vi "scanFrontPanel.vi"(8 "error in (no error)":errorcluster, 9 "index":i16, 10 "ScriptEventList":refnum<class "ScriptEventList.lvclass">, 11 "ScanCreator in":refnum<class "ScanCreator.lvclass">) -> (0 "error out":errorcluster, 1 "cancelled":bool, 2 "scriptListArray":refnum<class "ScriptEventList.lvclass">[](array[class]), 3 "ScanCreator out":refnum<class "ScanCreator.lvclass">, 4 "scanType":string, 5 "Values":string[](array[string]))   [LabVIEW 2011, in "Views.lvlib" / "ScriptEditor.lvlib" / "ScanCreator.lvclass"]
uses:
  ScanCreator.lvclass
  Tools/Scripting/ScriptingEvent/ScriptEventList/ScriptEventList.lvclass
  ScanCreator.lvclass/ScanCreator.ctl
panel:
  in  "Steps":dbl
  in  "Cancel":bool
  in  "ok":bool
  in  "Delay All?":bool=TRUE
  in  "Increment":dbl
  in  "EndValue":dbl format="%#_8g"
  in  "StartValue":dbl format="%#.8g"
  in  "Scan Type":u16(ring) items=["Time", "Time Difference", "Start Value", "End Value", "Step Value", "Ramp Time"]
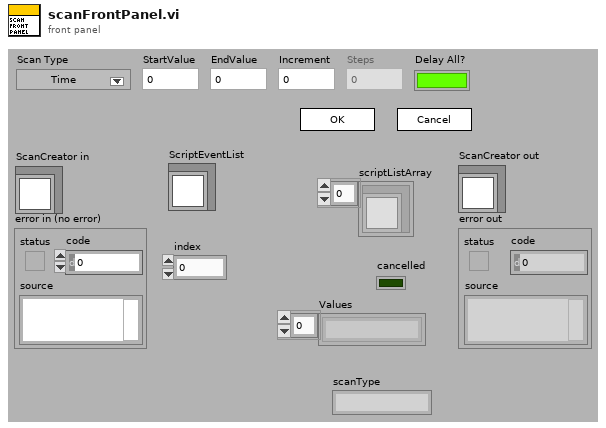
[diagram p1: front panel]
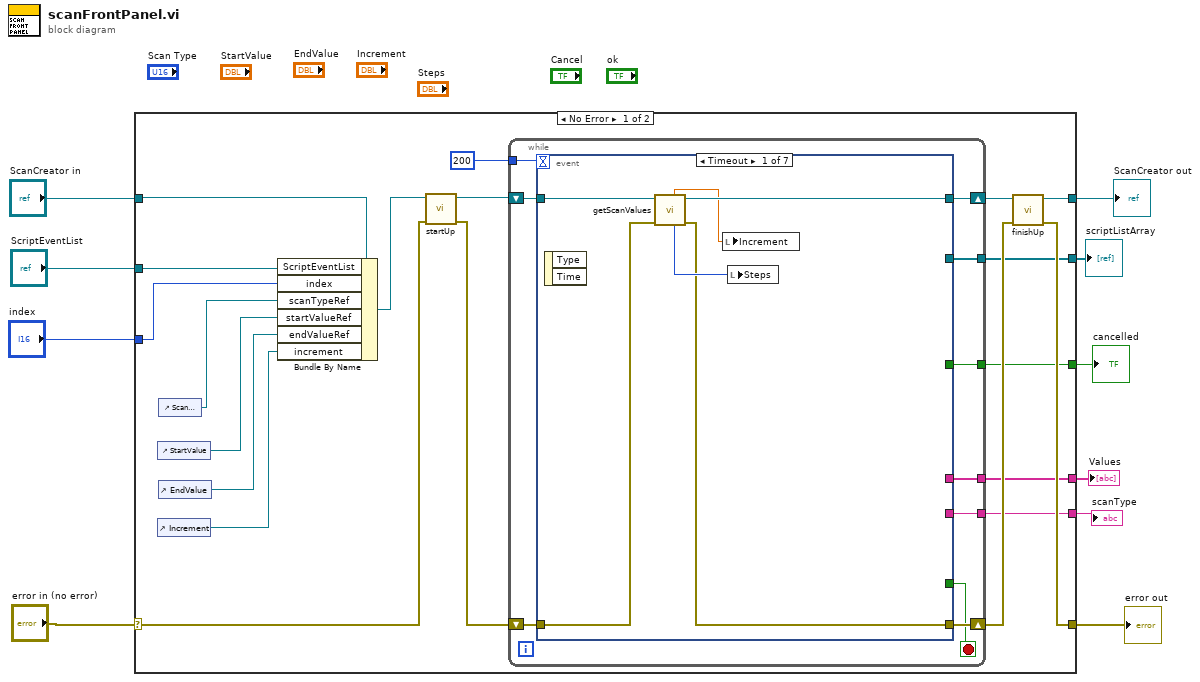
[diagram p0: block diagram]
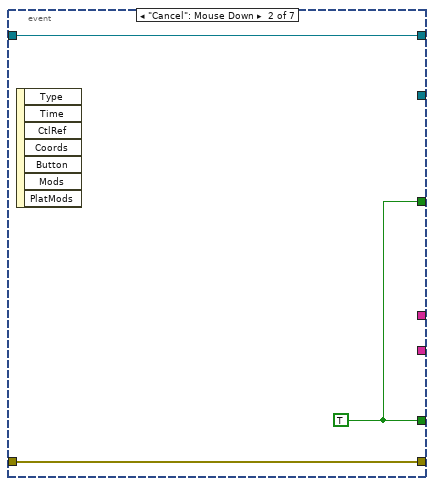
[diagram p2: hidden frame]
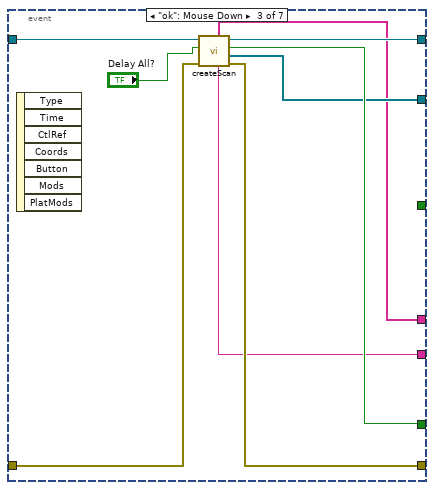
[diagram p3: hidden frame]
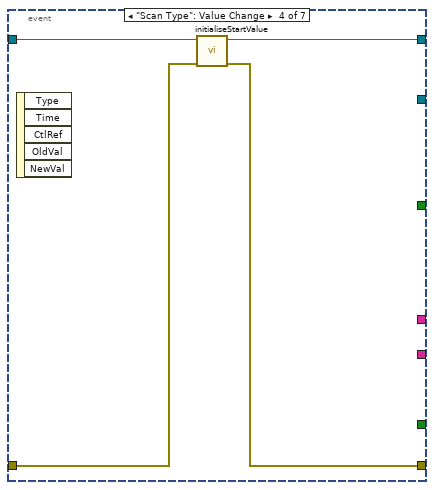
[diagram p4: hidden frame]
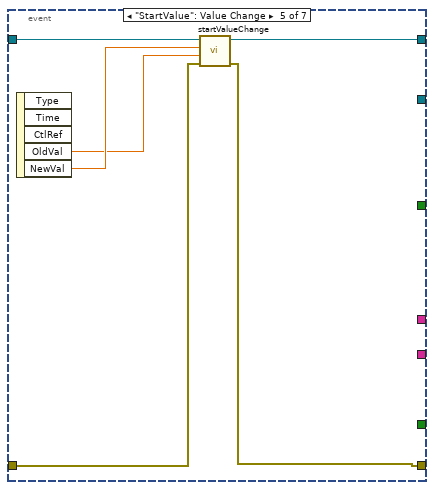
[diagram p5: hidden frame]
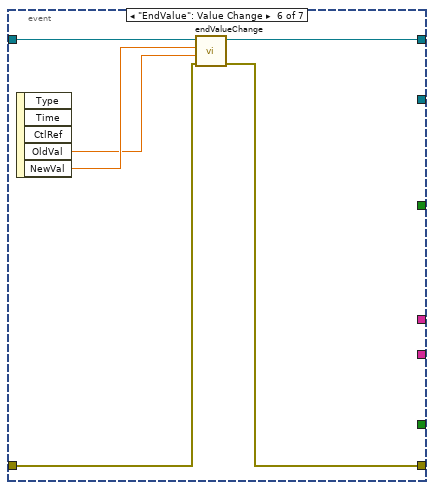
[diagram p6: hidden frame]
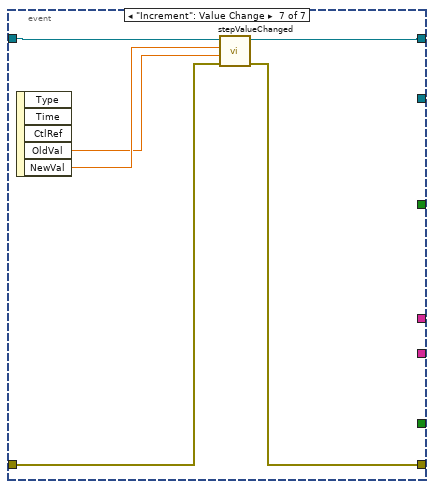
[diagram p7: hidden frame]
diagram:
  n1 = case shown="No Error" "error in (no error)" {
    selector: "error in (no error)" -> [w29 w82]
    tunnel: [w24 w82] -> w9
    tunnel: [w26 w81] -> w7
    tunnel: "ScanCreator in" -> [w19 w81]
    tunnel: "ScriptEventList" -> [w23 _]
    tunnel: "index" -> [w22 _]
    tunnel: [w17 _] -> w4
    tunnel: [w16 _] -> w3
    tunnel: [w15 _] -> w2
    tunnel: [w14 _] -> w1
    frame No Error {
      n2 = control-ref of="StartValue"() -> (w21:refnum<vi>)
      n3 = control-ref of="Increment"() -> (w20:refnum<vi>)
      n4 = control-ref of="Scan Type"() -> (w12:refnum<vi>)
      n5 = control-ref of="EndValue"() -> (w13:refnum<vi>)
      n6 = Bundle By Name(cluster=w19, "ScriptEventList"=w23, "index"=w22, "scanTypeRef"=w12, "startValueRef"=w21, "endValueRef"=w13, "increment"=w20) -> (w18:refnum<class "ScanCreator.lvclass">)
      n7 = call "startUp.vi"("error in (no error)"=w29, "ScanCreator in"=w18) -> ("error out"=w28:errorcluster, "ScanCreator out"=w30:refnum<class "ScanCreator.lvclass">)  [unwired: 8 in]
      n8 = while {
        shift-right: [w40] -> w25
        shift-left: w28 -> [w39]
        shift-right: [w38] -> w27
        shift-left: w30 -> [w37]
        tunnel: [w35] -> w17
        tunnel: [w34] -> w16
        tunnel: [w33] -> w15
        tunnel: [w32] -> w14
        tunnel: 200 -> [w31]
        stop <- w36 stop-if-true
        n9 = event shown="[0] Timeout" {
          selector: _ -> [_ _ _ _ _ _ _]
          dyn-events: _ -> [_ _ _ _ _ _ _]
          timeout: w31 -> [_ _ _ _ _ _ _]
          tunnel: [w41 w48 w56 w59 w65 w72 w75] -> w40
          tunnel: w39 -> [w42 w48 w57 w60 w66 w71 w76]
          tunnel: [w45 w49 w55 w61 w67 w73 w79] -> w38
          tunnel: w37 -> [w46 w49 w58 w62 w68 w74 w80]
          tunnel: [_ w47 w54 _ _ _ _] -> w36
          tunnel: [_ _ w52 _ _ _ _] -> w35
          tunnel: [_ w47 _ _ _ _ _] -> w34
          tunnel: [_ _ w51 _ _ _ _] -> w33
          tunnel: [_ _ w50 _ _ _ _] -> w32
          event Timeout {
            n10 = event-data() -> ()  [unwired: 1 in, 2 out]
            n11 = call "getScanValues.vi"("error in (no error)"=w42, "ScanCreator in"=w46) -> ("error out"=w41:errorcluster, "ScanCreator out"=w45:refnum<class "ScanCreator.lvclass">, "step"=w43:i16, "increment"=w44:dbl)  [unwired: 4 in, 2 out]
            n12 = local write "Increment"(w44) -> ()
            n13 = local write "Steps"(w43) -> ()
          }
          event "Cancel": Mouse Down {
            w47 = TRUE
            n14 = event-data() -> ()  [unwired: 1 in, 7 out]
          }
          event "ok": Mouse Down {
            n15 = event-data() -> ()  [unwired: 1 in, 7 out]
            n16 = call "createScan.vi"("error in (no error)"=w57, "delayAll"="Delay All?", "ScanCreator in"=w58) -> ("error out"=w56:errorcluster, "scriptListArray"=w52:refnum<class "ScriptEventList.lvclass">[], "close"=w54:bool, "ScanCreator out"=w55:refnum<class "ScanCreator.lvclass">, "scanType"=w50:string, "Values"=w51:string[])  [unwired: 3 in]
          }
          event "Scan Type": Value Change {
            n17 = event-data() -> ()  [unwired: 1 in, 5 out]
            n18 = call "initialiseStartValue.vi"("error in (no error)"=w60, "ScanCreator in"=w62) -> ("error out"=w59:errorcluster, "ScanCreator out"=w61:refnum<class "ScanCreator.lvclass">)  [unwired: 8 in]
          }
          event "StartValue": Value Change {
            n19 = event-data() -> ("OldVal"=w63:dbl, "NewVal"=w64:dbl)  [unwired: 1 in, 3 out]
            n20 = call "startValueChange.vi"("error in (no error)"=w66, "oldValue"=w63, "newValue"=w64, "ScanCreator in"=w68) -> ("error out"=w65:errorcluster, "ScanCreator out"=w67:refnum<class "ScanCreator.lvclass">)  [unwired: 6 in]
          }
          event "EndValue": Value Change {
            n21 = event-data() -> ("OldVal"=w69:dbl, "NewVal"=w70:dbl)  [unwired: 1 in, 3 out]
            n22 = call "endValueChange.vi"("error in (no error)"=w71, "oldValue"=w69, "newValue"=w70, "ScanCreator in"=w74) -> ("error out"=w72:errorcluster, "ScanCreator out"=w73:refnum<class "ScanCreator.lvclass">)  [unwired: 6 in]
          }
          event "Increment": Value Change {
            n23 = event-data() -> ("OldVal"=w77:dbl, "NewVal"=w78:dbl)  [unwired: 1 in, 3 out]
            n24 = call "stepValueChanged.vi"("error in (no error)"=w76, "oldValue"=w77, "newValue"=w78, "ScanCreator in"=w80) -> ("error out"=w75:errorcluster, "ScanCreator out"=w79:refnum<class "ScanCreator.lvclass">)  [unwired: 5 in, 1 out]
          }
        }
      }
      n25 = call "finishUp.vi"("error in (no error)"=w25, "ScanCreator in"=w27) -> ("error out"=w24:errorcluster, "ScanCreator out"=w26:refnum<class "ScanCreator.lvclass">)  [unwired: 8 in]
    }
    frame Error {
    }
  }
  "error out" <- w9
  "ScanCreator out" <- w7
  "scriptListArray" <- w4
  "cancelled" <- w3
  "Values" <- w2
  "scanType" <- w1
